vi "test_Format String to Numeric_Hexadecimal format.vi"(8 "error in (no error)":errorcluster, 11 "TestCase in":refnum<class "Instrument Addon Unit Tests.lvclass">) -> (0 "error out":errorcluster, 3 "TestCase out":refnum<class "Instrument Addon Unit Tests.lvclass">)   [LabVIEW 2018, in "Instrument Addon Unit Tests.lvclass"]
uses:
  Instrument Addon Unit Tests.lvclass
  Addon/Addon Shared/Types/Endian.ctl
  Addon/Addon Shared/Types/Data Channel Type.ctl
  <vilib>/addons/_JKI Toolkits/VI Tester/TestCase.llb/TestCase.lvclass
  Addon/Addon Engine/Instrument Addon Engine.lvlib
  Addon/Addon Shared/Instrument Addon Shared.lvlib
  C:/Program Files (x86)/National Instruments/LabVIEW 2018/vi.lib/addons/_JKI Toolkits/VI Tester/TestCase.llb/TestCase.lvclass
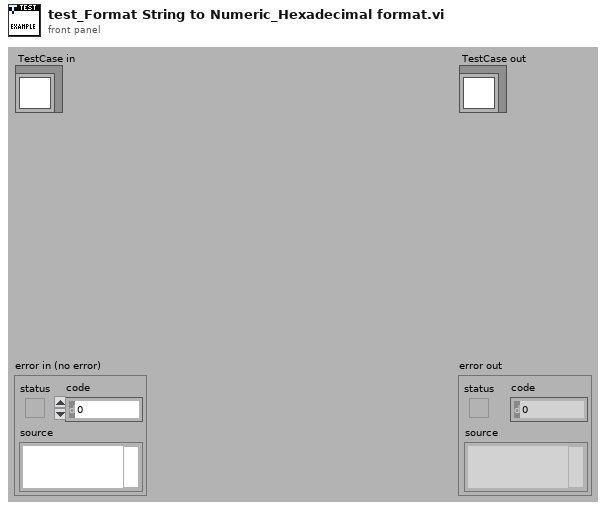
[diagram p1: front panel]
types:
  T1 = typedef "Instrument Addon Shared.lvlib/Data Channel Type.ctl" = enum16{"Format", "Comparison", "Type Cast", "Enumerated List"}
  T2 = typedef "Instrument Addon Shared.lvlib/Endian.ctl" = enum16{"Native", "Little", "Big"}
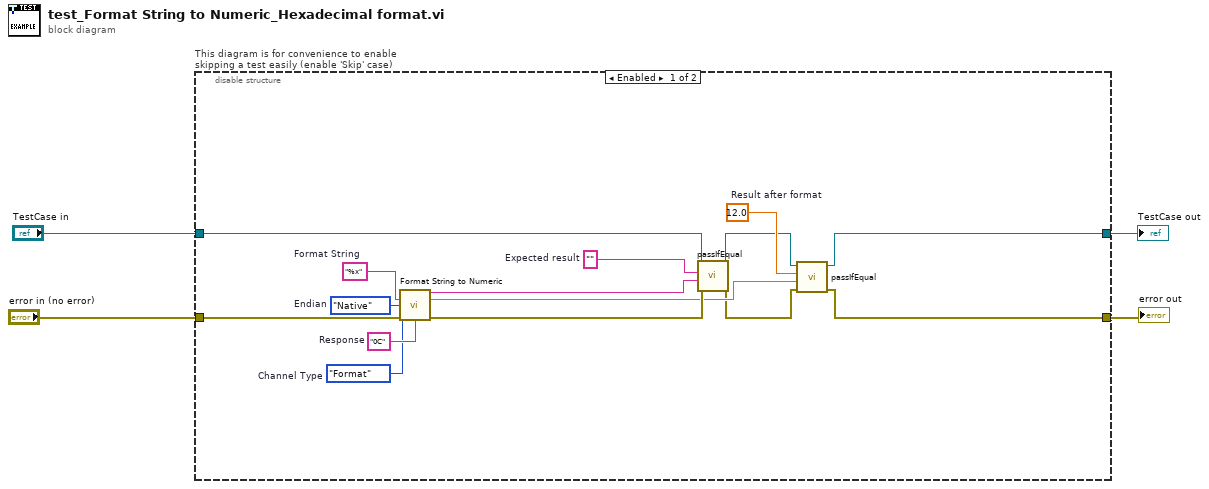
[diagram p0: block diagram]
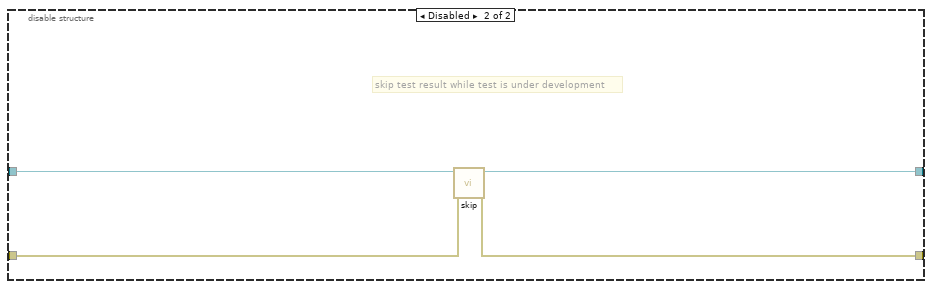
[diagram p2: hidden frame]
diagram:
  n1 = disable-structure "This diagram is for convenience to enable skipping a test easily (enable 'Skip' case)" shown="Enabled" {
    disable-tunnel: "TestCase in" -> [w19 w23]
    disable-tunnel: [w6 w21] -> w1
    disable-tunnel: [w8 w22] -> w3
    disable-tunnel: "error in (no error)" -> [w18 w20]
    frame Enabled {
      w5 = "%x"  # Format String
      w10 = 12.0  # Result after format
      w12 = Data_Channel_Type."Format"  # Channel Type
      w13 = ""  # Expected result
      w15 = "0C"  # Response
      w16 = Endian."Native"  # Endian
      n2 = call "Format String to Numeric.vi"("Format String"=w5, "Endian"=w16, "Channel Type"=w12, "error in (no error)"=w18, "Response"=w15) -> ("remaining string"=w14:string, "Value"=w11:dbl, "error out"=w17:errorcluster)  [unwired: 8 in]
      n3 = call-dynamic "passIfEqual.vi"("error in (no error)"=w17, "y"=w14, "x"=w13, "TestCase in"=w19) -> ("error out"=w9:errorcluster, "TestCase out"=w7:refnum<class "Instrument Addon Unit Tests.lvclass">)  [unwired: 6 in]
      n4 = call-dynamic "passIfEqual.vi"("error in (no error)"=w9, "y"=w11, "x"=w10, "TestCase in"=w7) -> ("error out"=w8:errorcluster, "TestCase out"=w6:refnum<class "Instrument Addon Unit Tests.lvclass">)  [unwired: 6 in]
    }
    frame Disabled {
      # "skip test result while test is under development"
      n5 = call <vilib>:"skip.vi"("error in (no error)"=w20, "TestCase in"=w23) -> ("error out"=w22:errorcluster, "TestCase out"=w21:refnum<class "Instrument Addon Unit Tests.lvclass">)  [unwired: 8 in]
    }
  }
  "error out" <- w3
  "TestCase out" <- w1
